vi "Init Sync Stuff.vi"(8 "error in (no error)":errorcluster, 10 "Dual Relay Bricklet in":refnum<class "Dual Relay Bricklet.lvclass">) -> (0 "error out":errorcluster, 2 "Dual Relay Bricklet out":refnum<class "Dual Relay Bricklet.lvclass">)   [LabVIEW 2011, in "Tinkerforge.lvlib" / "Dual Relay Bricklet.lvclass"]
doc: "This VI is the child implementation of \"Init Sync Stuff.vi\" and initializes all synchronization objects of this child object."
uses:
  Dual Relay Bricklet.lvclass
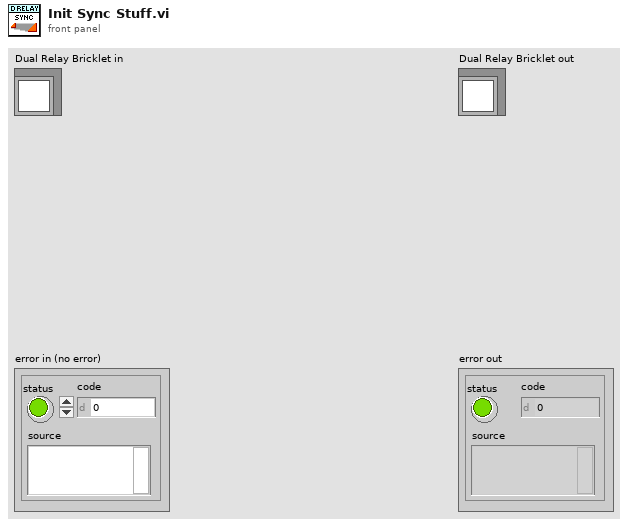
[diagram p1: front panel]
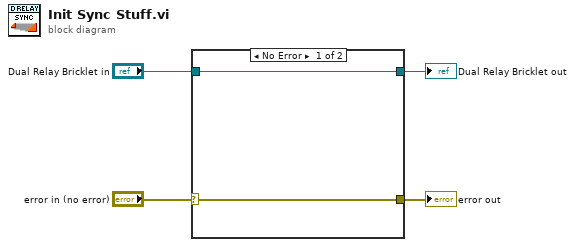
[diagram p0: block diagram]
diagram:
  n1 = case shown="No Error" "error in (no error)" {
    selector: "error in (no error)" -> [w5 w7]
    tunnel: "Dual Relay Bricklet in" -> [w6 w8]
    tunnel: [w5 w7] -> w2
    tunnel: [w6 w8] -> w1
    frame No Error {
    }
    frame Error {
    }
  }
  "error out" <- w2
  "Dual Relay Bricklet out" <- w1
